vi "New Layout.vi"(4 "PlotPane":refnum<vi>, 6 "Subpanel Refs (ALL)":refnum<vi>[](array[refnum]), 7 "RocketPlotPanel Type":refnum<class "RocketPlotPanel.lvclass">, 8 "error in (no error)":errorcluster, 10 "Layout":T6[](array[typedef]) {"Plot Bounds (%)"."Bottom (%)" format="%.2f"; "Plot Bounds (%)"."Top (%)" format="%.2f"; "Plot Bounds (%)"."Right (%)" format="%.2f"; "Plot Bounds (%)"."Left (%)" format="%.2f"}, 11 "Loop data in":T1 {"PanelMap"."Data"."Plot Bounds (%)"."Bottom (%)" format="%.2f"; "PanelMap"."Data"."Plot Bounds (%)"."Top (%)" format="%.2f"; "PanelMap"."Data"."Plot Bounds (%)"."Right (%)" format="%.2f"; "PanelMap"."Data"."Plot Bounds (%)"."Left (%)" format="%.2f"}) -> (0 "error out":errorcluster, 3 "Loop data out":T1 {"PanelMap"."Data"."Plot Bounds (%)"."Bottom (%)" format="%.2f"; "PanelMap"."Data"."Plot Bounds (%)"."Top (%)" format="%.2f"; "PanelMap"."Data"."Plot Bounds (%)"."Right (%)" format="%.2f"; "PanelMap"."Data"."Plot Bounds (%)"."Left (%)" format="%.2f"})   [LabVIEW 2021, in "MultiStokePlot.lvlib" / "MultiPlotPanel.lvclass"]
uses:
  Classes/MultiPlotPanel/MultiPlotPanel.lvclass
  Loop Data.ctl
  <vilib>/IlluminatedG/IG OOPanel/OOPanel/Manager/Manager.lvclass
  Panel Map.ctl
  Panel Map Data.ctl
  <userlib>/bjustice/RocketPlot/Classes/RocketPlotPanel/RocketPlotPanel.lvclass
  C:/Program Files/National Instruments/LabVIEW 2021/vi.lib/IlluminatedG/IG OOPanel/OOPanel/Panel/Panel.lvclass
  Window Position.ctl
  <vilib>/IlluminatedG/IG OOPanel/OOPanel/Panel/Panel Events.ctl
  <vilib>/IlluminatedG/IG OOPanel/OOPanel/Panel/Visbility Event Data.ctl
  <vilib>/IlluminatedG/IG OOPanel/OOPanel/Visibility State.ctl
  <vilib>/IlluminatedG/IG OOPanel/OOPanel/Close Reason.ctl
  Window Position and plot number.ctl
  <vilib>/Utility/miscctls.llb/LVMapReplaceAction.ctl
  <vilib>/IlluminatedG/IG OOPanel/OOPanel/OOPanel.lvlib
  <vilib>/IlluminatedG/IG OOPanel/OOPanel/Panel/Panel.lvclass
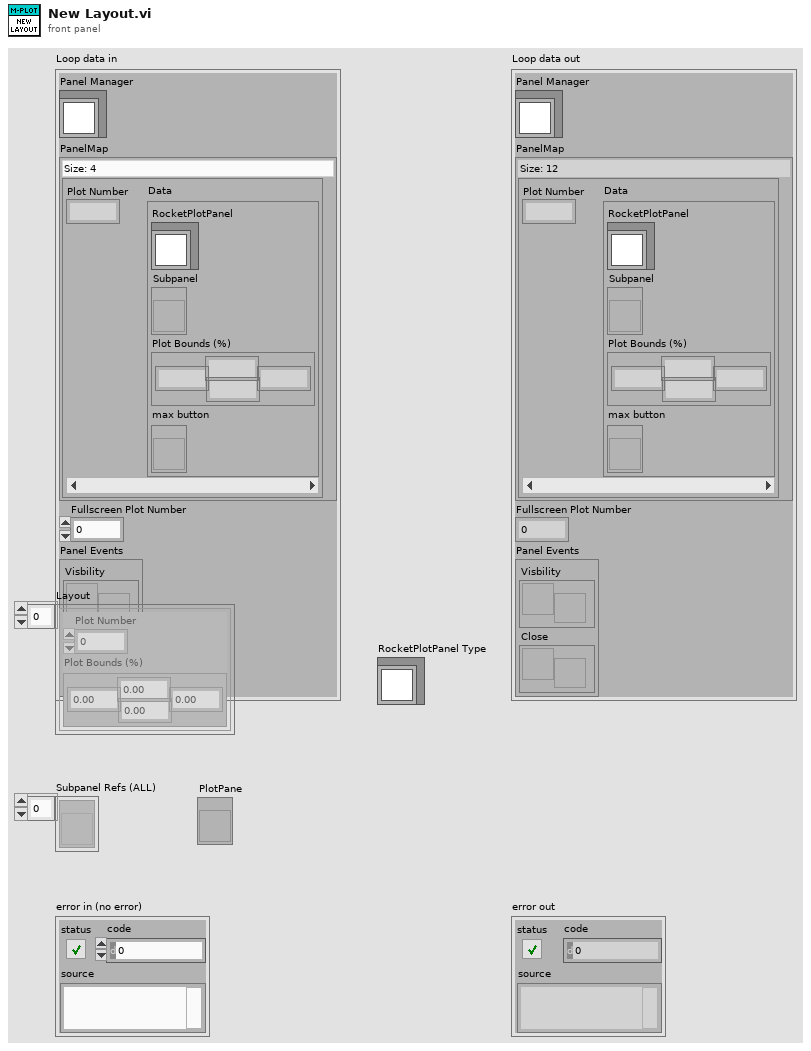
[diagram p1: front panel]
types:
  T1 = typedef "MultiStokePlot.lvlib/MultiPlotPanel.lvclass/Loop Data.ctl" = cluster{"Panel Manager":refnum<class "Manager.lvclass">, "PanelMap":T2, "Fullscreen Plot Number":i32, "Panel Events":T5}
  T2 = typedef "MultiStokePlot.lvlib/MultiPlotPanel.lvclass/Panel Map.ctl" = map{i32, T3}
  T3 = typedef "MultiStokePlot.lvlib/MultiPlotPanel.lvclass/Panel Map Data.ctl" = cluster{"RocketPlotPanel":refnum<class "RocketPlotPanel.lvclass">, "Subpanel":refnum<vi>, "Plot Bounds (%)":T4, "max button":refnum<vi>}
  T4 = typedef "MultiStokePlot.lvlib/MultiPlotPanel.lvclass/Window Position.ctl" = cluster{"Left (%)":dbl, "Top (%)":dbl, "Right (%)":dbl, "Bottom (%)":dbl}
  T5 = typedef "OOPanel.lvlib/Panel.lvclass/Panel Events.ctl" = cluster{"Visbility":refnum<user-event>, "Close":refnum<user-event>}
  T6 = typedef "MultiStokePlot.lvlib/MultiPlotPanel.lvclass/Window Position and plot number.ctl" = cluster{"Plot Number":i32, "Plot Bounds (%)":T4}
  T7 = typedef "LVMapReplaceAction.ctl" = enum32{"Modify Entry only if found", "Add or Modify Entry", "Delete Entry"}
  T8 = typedef "LVRectTypeDef.ctl" = cluster{"Left":i16, "Top":i16, "Right":i16, "Bottom":i16}
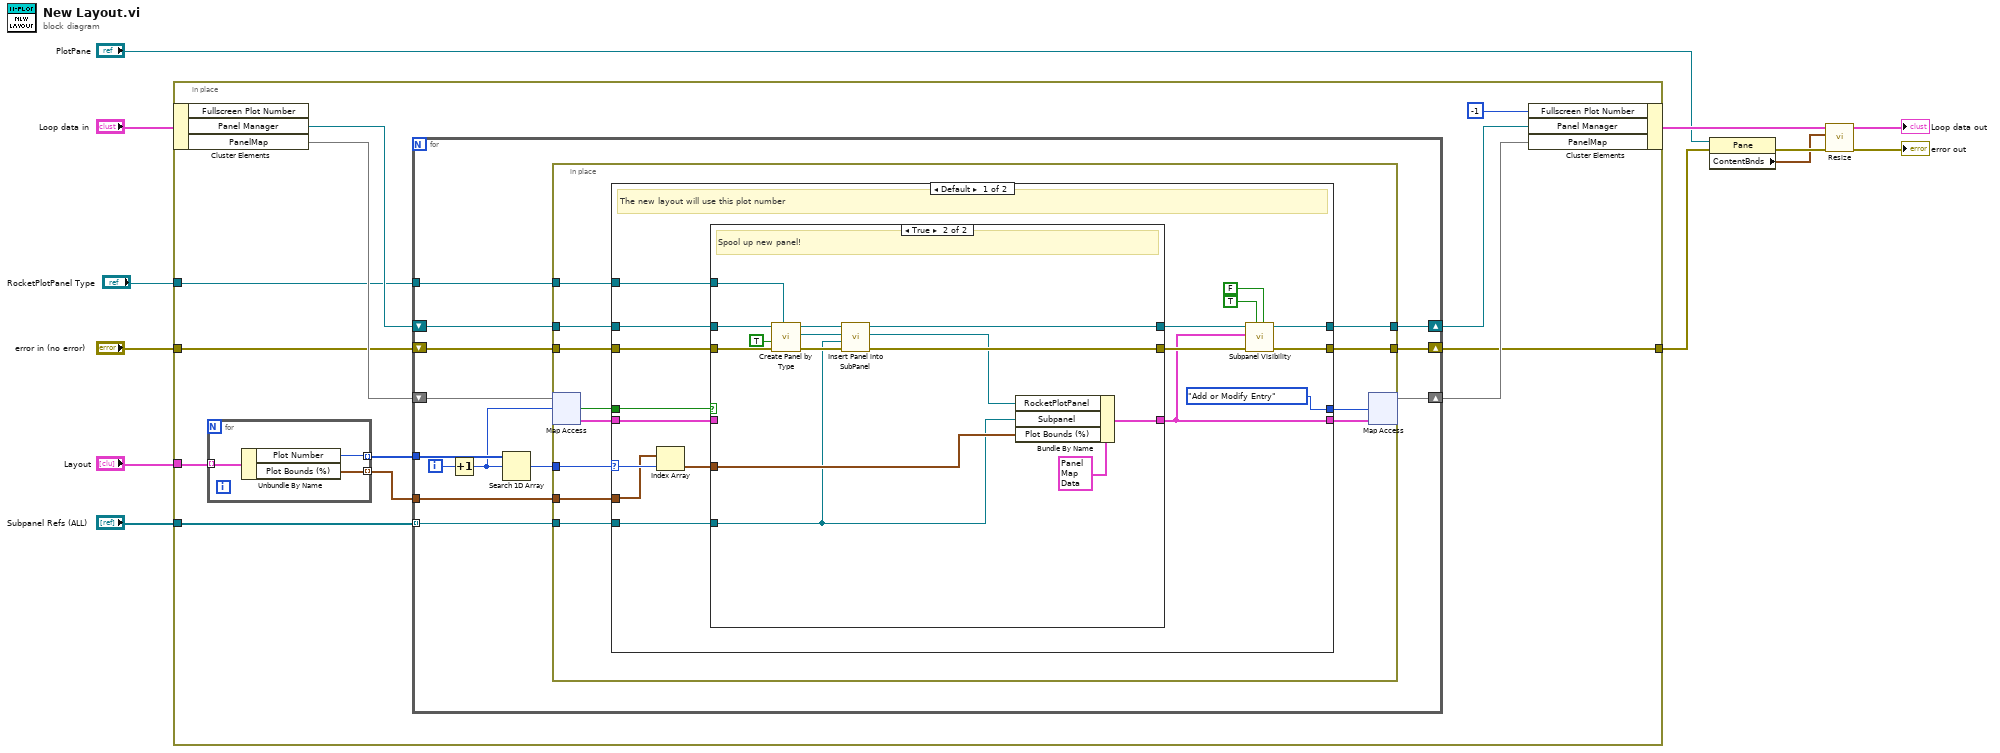
[diagram p0: block diagram]
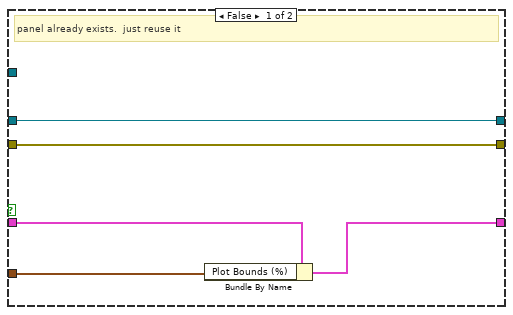
[diagram p2: hidden frame]
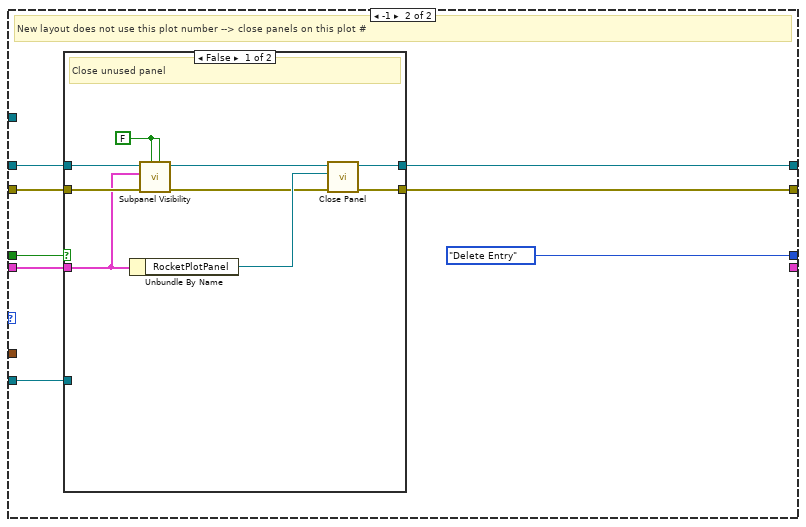
[diagram p3: hidden frame]
diagram:
  n1 = in-place {
    in-place-border: "Layout" -> [w18]
    in-place-border: "Subpanel Refs (ALL)" -> [w24]
    in-place-border: "error in (no error)" -> [w20]
    in-place-border: "RocketPlotPanel Type" -> [w16]
    in-place-border: [w13] -> w1
    n2 = in-place-cluster #1("Loop data in") -> ("Panel Manager"=w21:refnum<class "Manager.lvclass">, "PanelMap"=w22:T2)  [unwired: 1 out]
    n3 = for {
      tunnel: w18 -> [w27] mode=indexing
      tunnel: [w26] -> w23 mode=indexing
      tunnel: [w25] -> w17 mode=indexing
      n4 = Unbundle By Name(w27) -> ("Plot Number"=w26:i32, "Plot Bounds (%)"=w25:T4)
    }
    n5 = for {
      tunnel: w24 -> [w39] mode=indexing
      tunnel: w23 -> [w40]
      shift-right: [w37] -> w19
      shift-left: w22 -> [w38]
      shift-right: [w35] -> w14
      shift-left: w21 -> [w36]
      shift-right: [w32] -> w13
      shift-left: w20 -> [w33]
      tunnel: w17 -> [w31]
      tunnel: w16 -> [w28]
      i -> [w30]
      n6 = Increment(x=w30) -> (x+1=w29:i32)
      n7 = Search 1D Array(1D array=w40, element=w29) -> (index of element=w34:i32)  [unwired: 1 in]
      n8 = in-place {
        in-place-border: w39 -> [w43]
        in-place-border: w36 -> [w51]
        in-place-border: [w50] -> w35
        in-place-border: w34 -> [w47]
        in-place-border: w33 -> [w45]
        in-place-border: [w44] -> w32
        in-place-border: w31 -> [w42]
        in-place-border: w28 -> [w41]
        n9 = in-place-map #2(w38, w29) -> (w49:T3, w48:bool)  [unwired: 1 in]
        n10 = case shown="Default" w47 {
          selector: w47 -> [w66 _]
          tunnel: [LVMapReplaceAction."Add or Modify Entry" ("action") LVMapReplaceAction."Delete Entry" ("action")] -> w52
          tunnel: w51 -> [w56 w94]
          tunnel: [w58 w93] -> w50
          tunnel: w49 -> [w67 w92]
          tunnel: w48 -> [w68 w91]
          tunnel: [w59 _] -> w46
          tunnel: w45 -> [w55 w90]
          tunnel: [w57 w89] -> w44
          tunnel: w43 -> [w62 w88]
          tunnel: w42 -> [w65 _]
          tunnel: w41 -> [w63 _]
          frame Default {
            # "The new layout will use this plot number"
            n11 = Index Array(array=w65, index=w66) -> (element=w64:T4)
            n12 = case shown="True" w68 {
              tunnel: w56 -> [w74 w87]
              tunnel: [w74 w77] -> w61
              tunnel: [w70 w82] -> w59
              tunnel: w67 -> [w72 _]
              tunnel: w55 -> [w73 w84]
              tunnel: [w73 w81] -> w60
              tunnel: w62 -> [_ w75]
              tunnel: w64 -> [w71 w85]
              tunnel: w63 -> [_ w80]
              frame False {
                # "panel already exists.  just reuse it"
                n13 = Bundle By Name(cluster=w72, "Plot Bounds (%)"=w71) -> (w70:T3)
              }
              frame True {
                # "Spool up new panel!"
                n14 = call <vilib>:"Create Panel by Type.vi"("Panel Type"=w80, "error in (no error)"=w84, "Run? (T)"=TRUE, "Manager in"=w87) -> ("error out"=w81:errorcluster, "Panel"=w78:refnum<class "RocketPlotPanel.lvclass">, "Manager out"=w79:refnum<class "Manager.lvclass">)  [unwired: 5 in]
                n15 = call <vilib>:"Insert Panel into SubPanel.vi"("SubPanel"=w75, "Panel In"=w78, "Manager in"=w79) -> ("Panel"=w76:refnum<class "RocketPlotPanel.lvclass">, "Manager out"=w77:refnum<class "Manager.lvclass">)  [unwired: 6 in, 1 out]
                n16 = Bundle By Name(cluster=T3 {"RocketPlotPanel"=refnum, "Subpanel"=refnum, "Plot Bounds (%)"={"Left (%)"=0.0, "Top (%)"=0.0, "Right (%)"=0.0, "Bottom (%)"=0.0}, "max button"=refnum} ("Cluster"), "RocketPlotPanel"=w76, "Subpanel"=w75, "Plot Bounds (%)"=w85) -> (w82:T3)
              }
            }
            n17 = call "Subpanel Visibility.vi"("Maximized?"=FALSE, "Visible"=TRUE, "error in (no error)"=w60, "Panel"=w59, "Manager in"=w61) -> ("error out"=w57:errorcluster, "Manager out"=w58:refnum<class "Manager.lvclass">)  [unwired: 5 in]
          }
          frame -1 {
            # "New layout does not use this plot number --> close panels on this plot #"
            n18 = case shown="False" w91 {
              tunnel: w94 -> [w101 w106]
              tunnel: [w104 w106] -> w93
              tunnel: w92 -> [w97 _]
              tunnel: w90 -> [w100 w105]
              tunnel: [w103 w105] -> w89
              tunnel: w88 -> [_ _]
              frame False {
                w96 = FALSE ("Visible")
                # "Close unused panel"
                n19 = Unbundle By Name(w97) -> ("RocketPlotPanel"=w102:refnum<class "RocketPlotPanel.lvclass">)
                n20 = call "Subpanel Visibility.vi"("Maximized?"=w96, "Visible"=w96, "error in (no error)"=w100, "Panel"=w97, "Manager in"=w101) -> ("error out"=w98:errorcluster, "Manager out"=w99:refnum<class "Manager.lvclass">)  [unwired: 5 in]
                n21 = call <vilib>:"Close Panel.vi"("error in (no error)"=w98, "Panel"=w102, "Manager in"=w99) -> ("error out"=w103:errorcluster, "Manager out"=w104:refnum<class "Manager.lvclass">)  [unwired: 7 in]
              }
              frame True {
                # "no change"
              }
            }
          }
        }
        n22 = in-place-map #2(w46, w52) -> (w37:T2)  [unwired: 2 out]
      }
    }
    n23 = in-place-cluster #1("Fullscreen Plot Number"=-1, "Panel Manager"=w14, "PanelMap"=w19) -> (w8:T1)
  }
  n24 = property on="Property Node" class="Pane"(reference="PlotPane", error in=w1) -> (error out=w5:errorcluster, "ContentBnds"=w4:T8)  [unwired: 1 out]
  n25 = call "Resize.vi"("error in (no error)"=w5, "Pane.Content Area Rect"=w4, "Loop data in"=w8) -> ("error out"=→"error out":errorcluster, "Loop data out"=→"Loop data out":T1)  [unwired: 7 in]
